vi "Category Manager.vi"(8 "error in (no error)":errorcluster, 11 "Budgetizer.lvclass":refnum<class "Budgetizer.lvclass">) -> (0 "error out":errorcluster, 3 "Budgetizer.lvclass":refnum<class "Budgetizer.lvclass">)   [LabVIEW 2018, in "Budgetizer.lvclass"]
uses:
  Budgetizer.lvclass
  Category/Category.lvclass
panel:
  in  "Rename":bool
  in  "Delete":bool
  in  "Close":bool
  in  "Add":bool
  in  "Category Name":string
  in  "Category Table":i32(listbox)
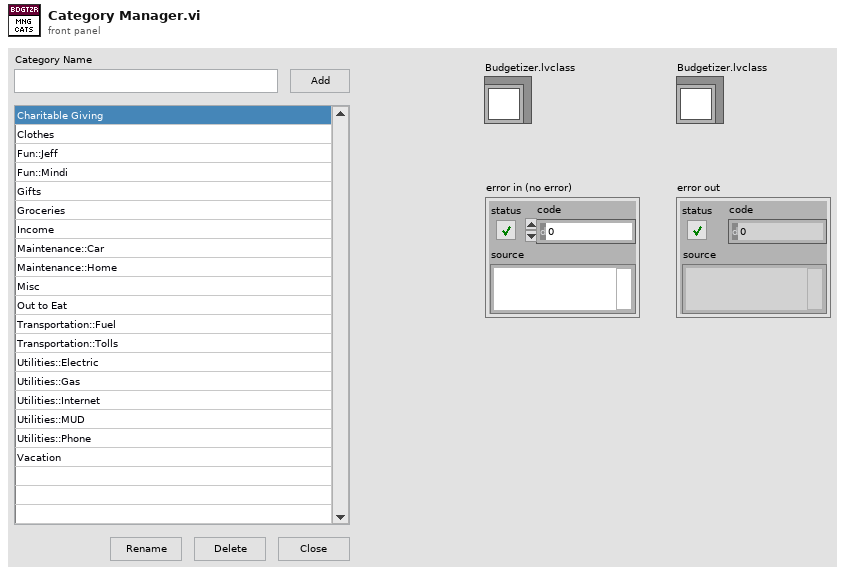
[diagram p1: front panel]
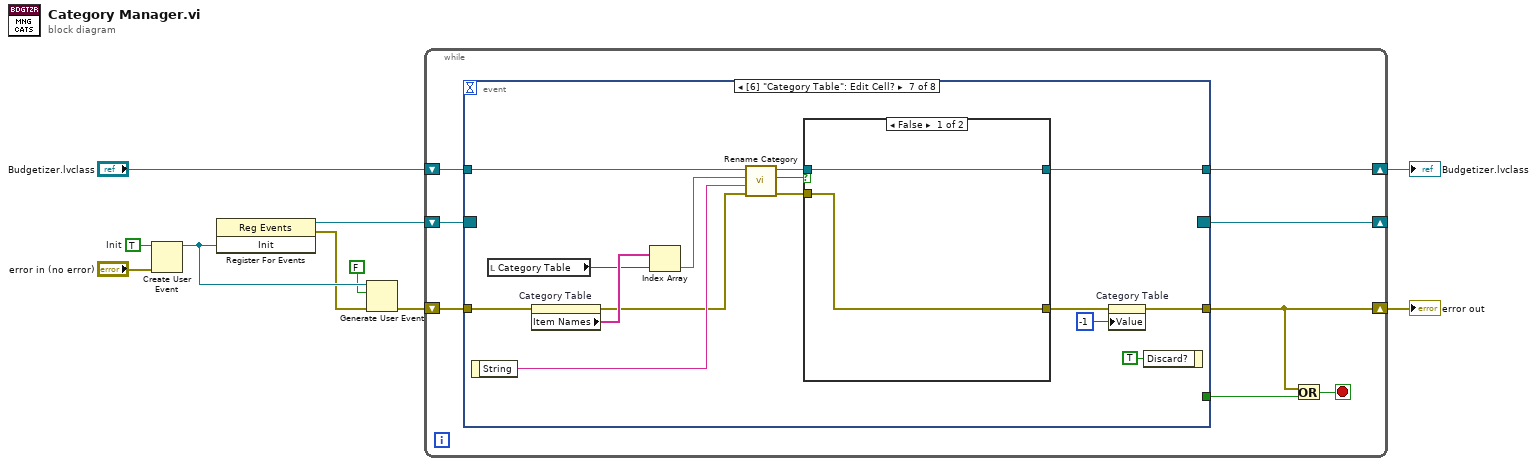
[diagram p0: block diagram]
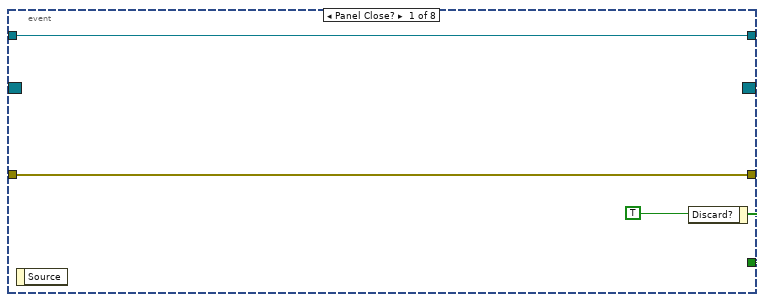
[diagram p2: hidden frame]
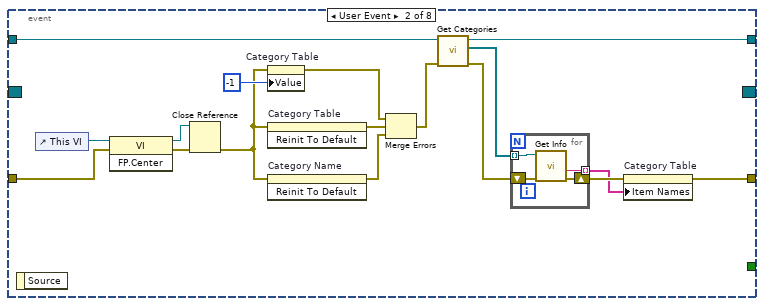
[diagram p3: hidden frame]
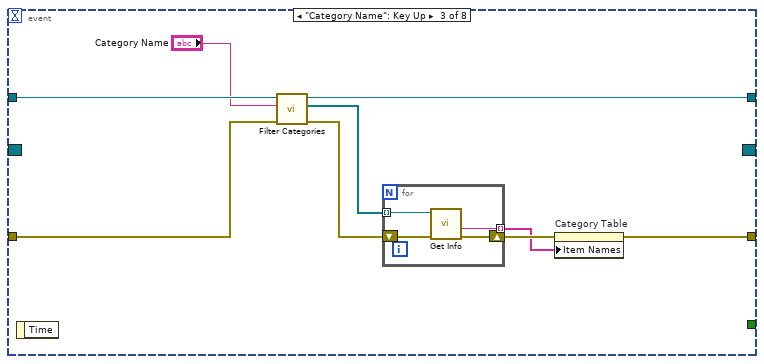
[diagram p4: hidden frame]
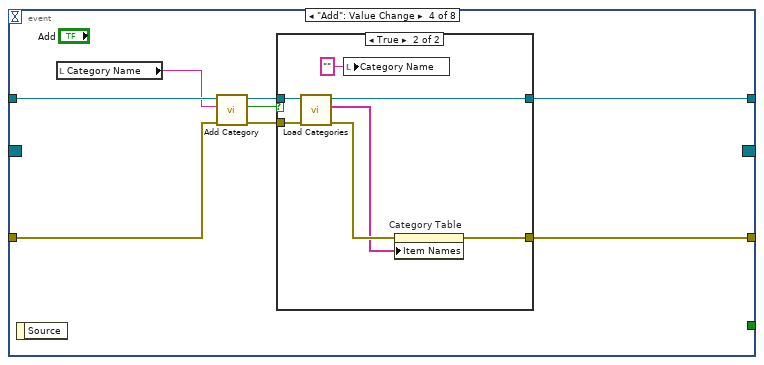
[diagram p5: hidden frame]
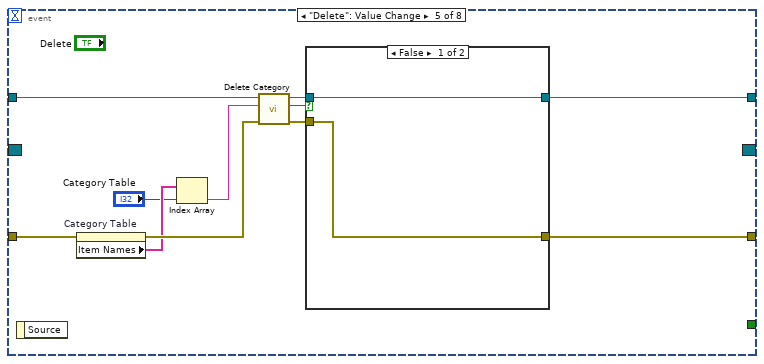
[diagram p7: hidden frame]
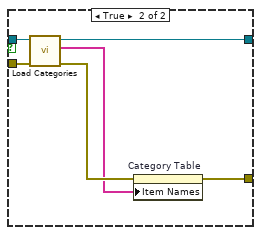
[diagram p8: hidden frame]
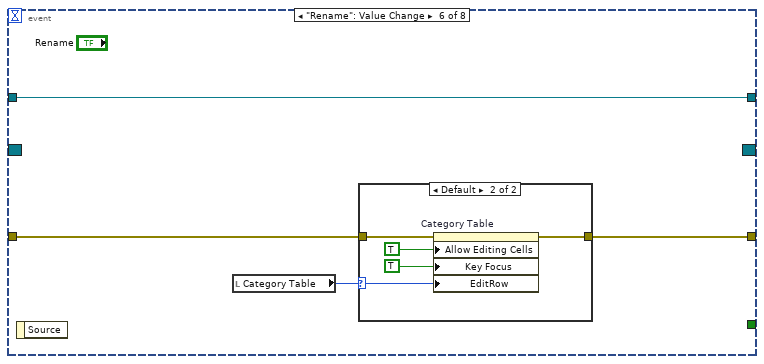
[diagram p9: hidden frame]
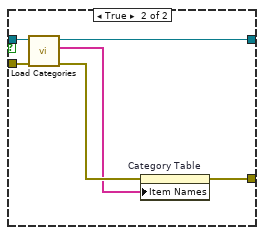
[diagram p11: hidden frame]
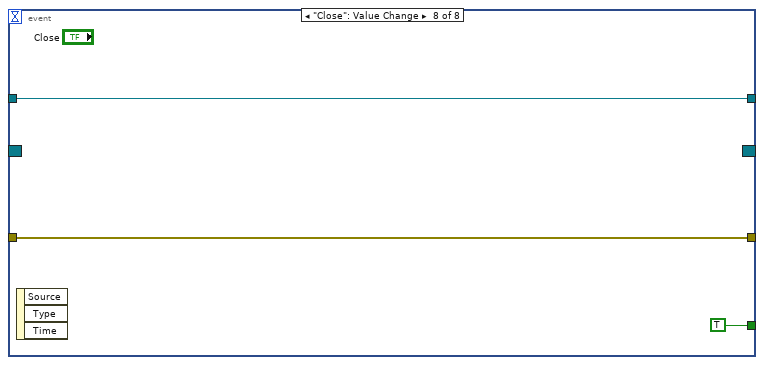
[diagram p12: hidden frame]
diagram:
  w10 = TRUE  # Init
  n1 = Create User Event(user event datatype=w10, error in="error in (no error)") -> (user event=w8:refnum<user-event>)  [unwired: 1 out]
  n2 = register-events(w8) -> (reference out=w9:refnum<event-registration>, error out=w7:errorcluster)  [unwired: 2 in]
  n3 = Generate User Event(user event=w8, event data cluster=FALSE ("event data"), error in=w7) -> (error out=w6:errorcluster)  [unwired: 1 in, 1 out]
  n4 = while {
    shift-right: [w16] -> _
    shift-left: w9 -> [w18]
    shift-right: [w13] -> w1
    shift-left: w6 -> [w17]
    shift-right: [w14] -> w2
    shift-left: "Budgetizer.lvclass" -> [w15]
    stop <- w11 stop-if-true
    n5 = event shown="[6] \"Category Table\": Edit Cell?" {
      selector: w18 -> [_ _ _ _ _ _ _ _]
      dyn-events: [_ _ _ _ _ _ _ _] -> w16
      timeout: _ -> [_ _ _ _ _ _ _ _]
      tunnel: [w21 _ _ _ _ _ _ TRUE ("Discard?")] -> w12
      tunnel: w17 -> [w20 w26 w51 w62 w82 w95 w114 w127]
      tunnel: [w20 w31 w43 w57 w76 w94 w102 w127] -> w13
      tunnel: w15 -> [w19 w28 w50 w63 w83 w93 w113 w126]
      tunnel: [w19 w38 w49 w58 w74 w93 w105 w126] -> w14
      event Panel Close? {
        w21 = TRUE ("Discard?")
        n6 = event-data() -> ()  [unwired: 1 in, 1 out]
        n7 = event-data("Discard?"=w21) -> ()  [unwired: 1 in, 1 out]
      }
      event User Event {
        n8 = event-data() -> ()  [unwired: 1 in, 1 out]
        n9 = control-ref of="This VI"() -> (w27:refnum<vi>)
        n10 = invoke class="VI" method="FP.Center"(reference=w27, error in=w26) -> (reference out=w24:refnum<vi>, error out=w25:errorcluster)  [unwired: 1 in, 1 out]
        n11 = Close Reference(reference=w24, error in (no error)=w25) -> (error out=w23:errorcluster)
        n12 = property on="Category Table" class="LstBox (strict)"(error in=w23, "Value"=-1 ("Category Table")) -> (error out=w22:errorcluster)  [unwired: 1 in, 1 out]
        n13 = invoke on="Category Table" class="LstBox (strict)" method="Reinit To Default"(error in=w23) -> (error out=w35:errorcluster)  [unwired: 2 in, 2 out]
        n14 = invoke on="Category Name" class="Str" method="Reinit To Default"(error in=w23) -> (error out=w36:errorcluster)  [unwired: 2 in, 2 out]
        n15 = Merge Errors(w22, w35, w36) -> (w34:errorcluster)
        n16 = call "Get Categories.vi"("error in (no error)"=w34, "Budgetizer in"=w28) -> ("error out"=w37:errorcluster, "All Categories"=w33:refnum<class "Category.lvclass">[], "Budgetizer out"=w38:refnum<class "Budgetizer.lvclass">)  [unwired: 7 in]
        n17 = for {
          tunnel: w33 -> [w42] mode=indexing
          shift-right: [w40] -> w32
          shift-left: w37 -> [w41]
          tunnel: [w39] -> w30 mode=indexing
          n18 = call "Get Info.vi"("error in (no error)"=w41, "Category in"=w42) -> ("error out"=w40:errorcluster, "Name"=w39:string)  [unwired: 6 in, 2 out]
        }
        n19 = property on="Category Table" class="LstBox (strict)"(error in=w32, "Item Names"=w30) -> (error out=w31:errorcluster)  [unwired: 1 in, 1 out]
      }
      event "Category Name": Key Up {
        n20 = event-data() -> ()  [unwired: 1 in, 1 out]
        n21 = call "Filter Categories.vi"("error in (no error)"=w51, "String Input"="Category Name", "Budgetizer in"=w50) -> ("error out"=w47:errorcluster, "Matching Categories"=w46:refnum<class "Category.lvclass">[], "Budgetizer out"=w49:refnum<class "Budgetizer.lvclass">)  [unwired: 6 in]
        n22 = for {
          tunnel: w46 -> [w55] mode=indexing
          shift-right: [w53] -> w45
          shift-left: w47 -> [w54]
          tunnel: [w52] -> w44 mode=indexing
          n23 = call "Get Info.vi"("error in (no error)"=w54, "Category in"=w55) -> ("error out"=w53:errorcluster, "Name"=w52:string)  [unwired: 6 in, 2 out]
        }
        n24 = property on="Category Table" class="LstBox (strict)"(error in=w45, "Item Names"=w44) -> (error out=w43:errorcluster)  [unwired: 1 in, 1 out]
      }
      event "Add": Value Change {
        n25 = event-data() -> ()  [unwired: 1 in, 1 out]
        n26 = local read "Category Name"() -> (w61:string)
        n27 = call "Add Category.vi"("error in (no error)"=w62, "Category Name"=w61, "Budgetizer in"=w63) -> ("error out"=w59:errorcluster, "Anything Added?"=w56:bool, "Budgetizer out"=w60:refnum<class "Budgetizer.lvclass">)  [unwired: 6 in]
        n28 = case shown="True" w56 {
          tunnel: w60 -> [w65 w72]
          tunnel: w59 -> [w64 w71]
          tunnel: [w65 w69] -> w58
          tunnel: [w64 w70] -> w57
          frame False {
          }
          frame True {
            n29 = call "Load Categories.vi"("error in (no error)"=w71, "Budgetizer in"=w72) -> ("error out"=w68:errorcluster, "Names Loaded"=w67:string[], "Budgetizer out"=w69:refnum<class "Budgetizer.lvclass">)  [unwired: 7 in]
            n30 = local write "Category Name"("" ("Category Name")) -> ()
            n31 = property on="Category Table" class="LstBox (strict)"(error in=w68, "Item Names"=w67) -> (error out=w70:errorcluster)  [unwired: 1 in, 1 out]
          }
        }
      }
      event "Delete": Value Change {
        n32 = event-data() -> ()  [unwired: 1 in, 1 out]
        n33 = property on="Category Table" class="LstBox (strict)"(error in=w82) -> (error out=w81:errorcluster, "Item Names"=w80:string[])  [unwired: 1 in, 1 out]
        n34 = Index Array(array=w80, index="Category Table") -> (element=w78:string)
        n35 = call "Delete Category.vi"("error in (no error)"=w81, "Category Name"=w78, "Budgetizer in"=w83) -> ("error out"=w77:errorcluster, "Anything Deleted?"=w73:bool, "Budgetizer out"=w75:refnum<class "Budgetizer.lvclass">)  [unwired: 6 in]
        n36 = case shown="False" w73 {
          tunnel: w75 -> [w85 w91]
          tunnel: w77 -> [w84 w90]
          tunnel: [w85 w88] -> w74
          tunnel: [w84 w89] -> w76
          frame False {
          }
          frame True {
            n37 = call "Load Categories.vi"("error in (no error)"=w90, "Budgetizer in"=w91) -> ("error out"=w87:errorcluster, "Names Loaded"=w86:string[], "Budgetizer out"=w88:refnum<class "Budgetizer.lvclass">)  [unwired: 7 in]
            n38 = property on="Category Table" class="LstBox (strict)"(error in=w87, "Item Names"=w86) -> (error out=w89:errorcluster)  [unwired: 1 in, 1 out]
          }
        }
      }
      event "Rename": Value Change {
        n39 = event-data() -> ()  [unwired: 1 in, 1 out]
        n40 = local read "Category Table"() -> (w92:i32)
        n41 = case shown="Default" w92 {
          selector: w92 -> [_ w97]
          tunnel: w95 -> [w96 w101]
          tunnel: [w96 w99] -> w94
          frame ..-1 {
          }
          frame Default {
            n42 = property on="Category Table" class="LstBox (strict)"(error in=w101, "Allow Editing Cells"=TRUE, "Key Focus"=TRUE, "EditRow"=w97) -> (error out=w99:errorcluster)  [unwired: 1 in, 1 out]
          }
        }
      }
      event "Category Table": Edit Cell? {
        n43 = event-data() -> ("String"=w112:string)  [unwired: 1 in]
        n44 = local read "Category Table"() -> (w115:i32)
        n45 = property on="Category Table" class="LstBox (strict)"(error in=w114) -> (error out=w110:errorcluster, "Item Names"=w116:string[])  [unwired: 1 in, 1 out]
        n46 = Index Array(array=w116, index=w115) -> (element=w111:string)
        n47 = call "Rename Category.vi"("error in (no error)"=w110, "New Name"=w112, "Old Name"=w111, "Budgetizer in"=w113) -> ("error out"=w106:errorcluster, "Anything Renamed?"=w107:bool, "Budgetizer out"=w108:refnum<class "Budgetizer.lvclass">)  [unwired: 5 in]
        n48 = case shown="False" w107 {
          tunnel: w108 -> [w118 w124]
          tunnel: w106 -> [w117 w123]
          tunnel: [w118 w122] -> w105
          tunnel: [w117 w119] -> w103
          frame False {
          }
          frame True {
            n49 = call "Load Categories.vi"("error in (no error)"=w123, "Budgetizer in"=w124) -> ("error out"=w121:errorcluster, "Names Loaded"=w120:string[], "Budgetizer out"=w122:refnum<class "Budgetizer.lvclass">)  [unwired: 7 in]
            n50 = property on="Category Table" class="LstBox (strict)"(error in=w121, "Item Names"=w120) -> (error out=w119:errorcluster)  [unwired: 1 in, 1 out]
          }
        }
        n51 = property on="Category Table" class="LstBox (strict)"(error in=w103, "Value"=-1 ("Category Table")) -> (error out=w102:errorcluster)  [unwired: 1 in, 1 out]
        n52 = event-data("Discard?"=TRUE) -> ()  [unwired: 1 in, 1 out]
      }
      event "Close": Value Change {
        n53 = event-data() -> ()  [unwired: 1 in, 3 out]
      }
    }
    n54 = Or(x=w13, y=w12) -> (x .or. y?=w11:bool)
  }
  "Budgetizer.lvclass" <- w2
  "error out" <- w1
